vi "Get Epoch Time.vi"(10 "Timestamp (now)":timestamp, 11 "Epoch (Local)":refnum<class "Epoch.lvclass">) -> (1 "Fractional Second":dbl format="%#.19f", 2 "Epoch Time (s)":i64, 3 "Epoch out":refnum<class "Epoch.lvclass">)   [LabVIEW 2021]
uses:
  epoch/Epoch.lvclass
  epoch/leapSeconds LUT.vi
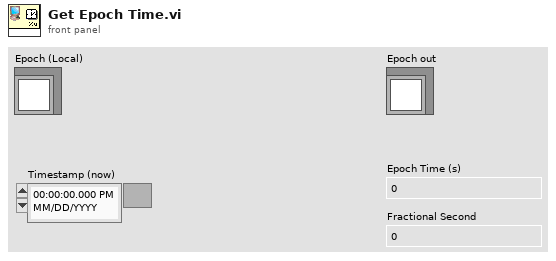
[diagram p1: front panel]
types:
  T1 = typedef "LVDateTimeRec.ctl" = cluster{"fractional second":dbl, "second":i32, "minute":i32, "hour":i32, "day of month":i32, "month":i32, "year":i32, "day of week":i32, "day of year":i32, "DST":i32}
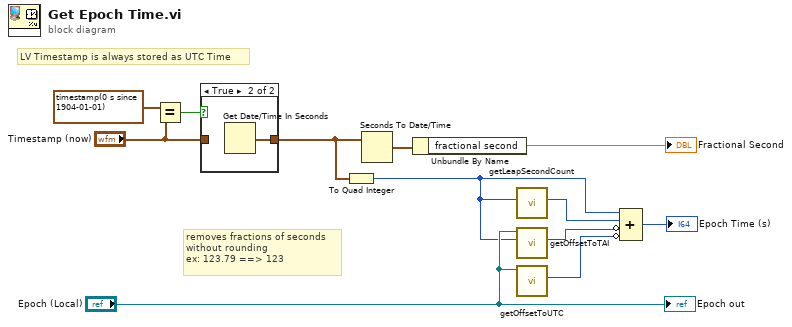
[diagram p0: block diagram]
diagram:
  # "LV Timestamp is always stored as UTC Time"
  # "removes fractions of seconds\nwithout rounding\nex: 123.79 ==> 123"
  n1 = Equal?(x=timestamp(0 s since 1904-01-01), y="Timestamp (now)") -> (x = y?=w11:bool)
  n2 = case shown="True" w11 {
    tunnel: [w13 w14] -> w3
    tunnel: "Timestamp (now)" -> [w13 _]
    frame False {
    }
    frame True {
      n3 = Get Date/Time In Seconds() -> (seconds since 1Jan1904=w14:timestamp)
    }
  }
  n4 = To Quad Integer(1:w3) -> (0:w6:i64)
  n5 = Seconds To Date/Time(time stamp (now)=w3) -> (date time rec=w2:T1)  [unwired: 1 in]
  n6 = Unbundle By Name(w2) -> ("fractional second"=→"Fractional Second":dbl)
  n7 = call "getLeapSecondCount.vi"("UTC Epoch Time"=w6) -> ("Leap Seconds"=w4:i64)  [unwired: 10 in]
  n8 = call-dynamic "getOffsetToTAI.vi"("Epoch Time"=w6, "Epoch"="Epoch (Local)") -> ("Offset to TAI"=w5:i64)  [unwired: 9 in]
  n9 = call-dynamic "getOffsetToUTC.vi"("Epoch"="Epoch (Local)") -> ("Offset to UTC"=w9:i64)  [unwired: 10 in]
  n10 = Compound Arithmetic op=ADD(w6, w4, invert w5, invert w9) -> (→"Epoch Time (s)":i64)
  "Epoch out" <- "Epoch (Local)"
